vi "sequencerGlobVarsWrite.vi"(0 "seqState":T1 caption="fpgaState", 2 "cmdByHost":T1=enum."idle", 3 "abort":bool, 4 "halt":bool, 5 "hostConfirmsHzOffsetIsSet":bool, 10 "writeOnlySeqState":bool, 11 "pause":bool) -> ()   [LabVIEW 2014]
uses:
  sequencerState.ctl
  <vilib>/rvi/Emulation/niFpgaSctlEmulationGetInTimedLoop.vi
  sequencerGlobVars.vi
  <vilib>/rvi/Emulation/niFpgaProcessEmulError.vi
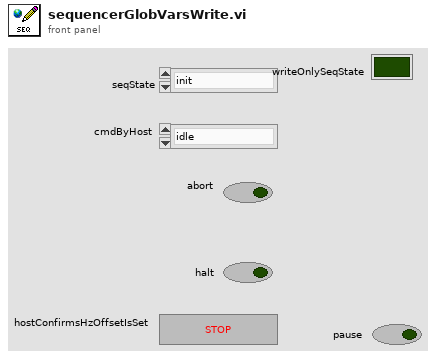
[diagram p1: front panel]
types:
  T1 = typedef "sequencerState.ctl" = enum16{"init", "idle", "measureOffset", "measureTrack", "measComplete", "error"}
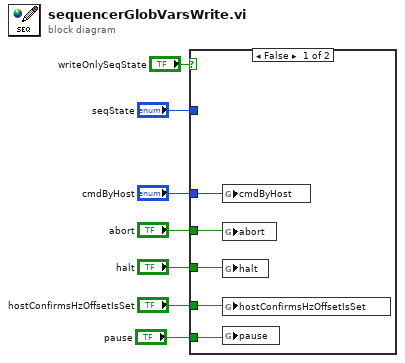
[diagram p0: block diagram]
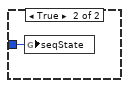
[diagram p2: hidden frame]
diagram:
  n1 = case shown="False" "writeOnlySeqState" {
    tunnel: "seqState" -> [_ w13]
    tunnel: "cmdByHost" -> [w12 _]
    tunnel: "abort" -> [w11 _]
    tunnel: "halt" -> [w10 _]
    tunnel: "hostConfirmsHzOffsetIsSet" -> [w9 _]
    tunnel: "pause" -> [w8 _]
    frame False {
      n2 = global write "sequencerGlobVars.vi" "cmdByHost"(w12) -> ()
      n3 = global write "sequencerGlobVars.vi" "abort"(w11) -> ()
      n4 = global write "sequencerGlobVars.vi" "halt"(w10) -> ()
      n5 = global write "sequencerGlobVars.vi" "hostConfirmsHzOffsetIsSet"(w9) -> ()
      n6 = global write "sequencerGlobVars.vi" "pause"(w8) -> ()
    }
    frame True {
      n7 = global write "sequencerGlobVars.vi" "seqState"(w13) -> ()
    }
  }
